vi "Get Size 2D.vi"(8 "error in (no error)":errorcluster, 11 "Abs_Array1D in":refnum<class "Abs_Array2D.lvclass">) -> (0 "error out":errorcluster, 1 "Column":i32, 2 "Row":i32, 3 "Abs_Array1D out":refnum<class "Abs_Array2D.lvclass">)   [LabVIEW 2021, in "Abs_Array2D.lvclass"]
uses:
  Abs_Array2D.lvclass
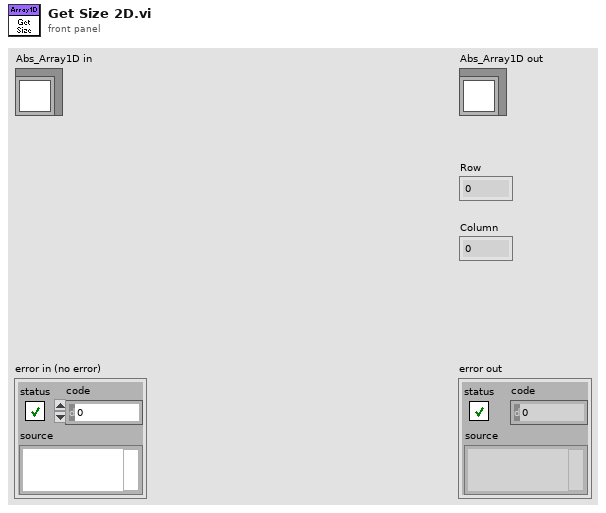
[diagram p1: front panel]
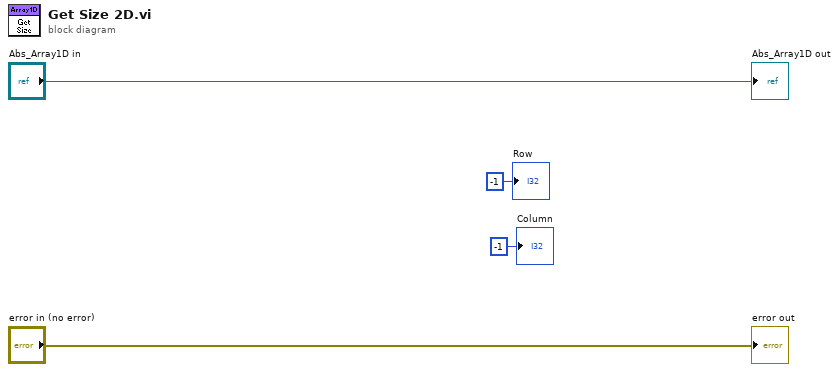
[diagram p0: block diagram]
diagram:
  "error out" <- "error in (no error)"
  "Abs_Array1D out" <- "Abs_Array1D in"
  "Row" <- -1 ("Size")
  "Column" <- -1 ("Column")
